vi "Export Markdown.vi"   [LabVIEW 2018]
doc: "Auto-generates markdown documentation from a LabVIEW Library.\n\nLaunches the <b>Tools > Export Markdown...</b>."
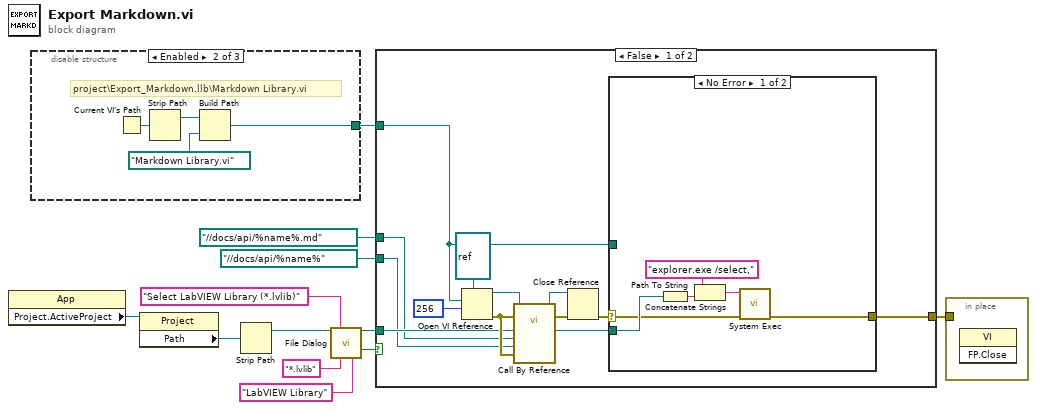
[diagram p0: block diagram]
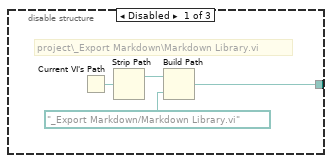
[diagram p2: hidden frame]
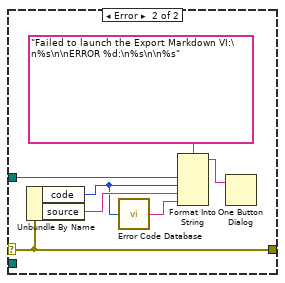
[diagram p4: hidden frame]
diagram:
  n1 = property class="App"() -> ("Project.ActiveProject"=w11:refnum<vi>)  [unwired: 2 in, 2 out]
  n2 = disable-structure shown="Enabled" {
    disable-tunnel: [w13 w17 _] -> w3
    frame Disabled {
      # "project\\_Export Markdown\\Markdown Library.vi"
      n3 = Current VI's Path() -> (path=w15:path)
      n4 = Strip Path(path=w15) -> (stripped path=w16:path)  [unwired: 1 out]
      n5 = Build Path(base path=w16, name or relative path=path "_Export Markdown/Markdown Library.vi") -> (appended path=w13:path)
    }
    frame Enabled {
      # "project\\Export_Markdown.llb\\Markdown Library.vi"
      n6 = Current VI's Path() -> (path=w19:path)
      n7 = Strip Path(path=w19) -> (stripped path=w20:path)  [unwired: 1 out]
      n8 = Build Path(base path=w20, name or relative path=path "Markdown Library.vi") -> (appended path=w17:path)
    }
    frame Disabled {
    }
  }
  n9 = property class="Project"(reference=w11) -> ("Path"=w10:path)  [unwired: 1 in, 2 out]
  n10 = Strip Path(path=w10) -> (stripped path=w9:path)  [unwired: 1 out]
  n11 = call "File Dialog"("start path"=w9, "prompt"="Select LabVIEW Library (*.lvlib)", "pattern (all files)"="*.lvlib", "pattern label"="LabVIEW Library") -> ("selected path"=w5:path, "cancelled"=w4:bool)  [unwired: 8 in, 2 out]
  n12 = case shown="False" w4 {
    tunnel: [w32 _] -> w12
    tunnel: w5 -> [w26 _]
    tunnel: w3 -> [w25 _]
    tunnel: path "../../docs/api/%name%.md" ("Markdown in (..\\..\\docs\\%name%.md)") -> [w22 _]
    tunnel: path "../../docs/api/%name%" ("Markdown Images Dir (..\\..\\docs\\%name%)") -> [w21 _]
    frame False {
      n13 = Open VI Reference(type specifier VI Refnum (for type only)=refnum<vi> refnum, vi path=w25, options=256) -> (vi reference=w29:refnum<vi>, error out=w28:errorcluster)  [unwired: 3 in]
      n14 = call-by-ref "?"(reference=w29, error in=w28, 8:"error in (no error)"=w28, "Markdown Images Dir (..\\..\\docs\\%name%)"=w21, "Markdown in (..\\..\\docs\\%name%.md)"=w22, "Library Path (*.lvlib)"=w26) -> (reference out=w27:refnum<vi>, error out=w30:errorcluster, "Markdown out"=w23:path)  [unwired: 5 in, 2 out]
      n15 = Close Reference(reference=w27, error in (no error)=w30) -> (error out=w33:errorcluster)
      n16 = case shown="No Error" w33 {
        selector: w33 -> [w35 w43]
        tunnel: w25 -> [_ w44]
        tunnel: [w34 w43] -> w32
        tunnel: w23 -> [w37 _]
        frame No Error {
          n17 = Path To String(path=w37) -> (string=w38:string)
          n18 = Concatenate Strings("explorer.exe /select,", w38) -> (w36:string)
          n19 = call <vilib>:"System Exec.vi"("error in (no error)"=w35, "command line"=w36) -> ("error out"=w34:errorcluster)  [unwired: 6 in, 3 out]
        }
        frame Error {
          n20 = Unbundle By Name(w43) -> ("code"=w42:i32, "source"=w46:string)
          n21 = call <vilib>:"Error Code Database.vi"("Error Code"=w42) -> ("Error Text"=w41:string)
          n22 = Format Into String(format string="Failed to launch the Export Markdown VI:\n%s\n\nERROR %d:\n%s\n\n%s", w44, w42, w46, w41) -> (resulting string=w40:string)  [unwired: 2 in, 1 out]
          n23 = One Button Dialog(message=w40) -> ()  [unwired: 1 in, 1 out]
        }
      }
    }
    frame True {
    }
  }
  n24 = in-place {
    in-place-border: w12 -> [_]
    n25 = invoke class="VI" method="FP.Close"() -> ()  [unwired: 3 in, 3 out]
  }
